vi "Write Outputs.vi"(8 "error in (no error)":errorcluster, 11 "Engine Data in":T1) -> (0 "error out":errorcluster, 3 "Engine Data out":T1)   [LabVIEW 2017, in "Routing and Faulting Engine.lvlib"]
uses:
  Routing and Faulting Engine.lvlib
  Engine Data.ctl
  Includes/CDMessaging.lvlibp/Producer/Abstract Producer/Abstract Producer.lvclass
  Shared/Compiled.Settings.ctl
  Shared/Communication Configuration.ctl
  Shared/Routing and Faulting Configuration.ctl
  Shared/Routing Channel Configuration.ctl
  Shared/Value-Connections Map.ctl
  Shared/Connection.ctl
  Shared/Alias Mapping.ctl
  Shared/FIFO Indices.ctl
  Device Inputs.ctl
  Device Outputs.ctl
  Shared/Routing and Faulting Shared.lvlib
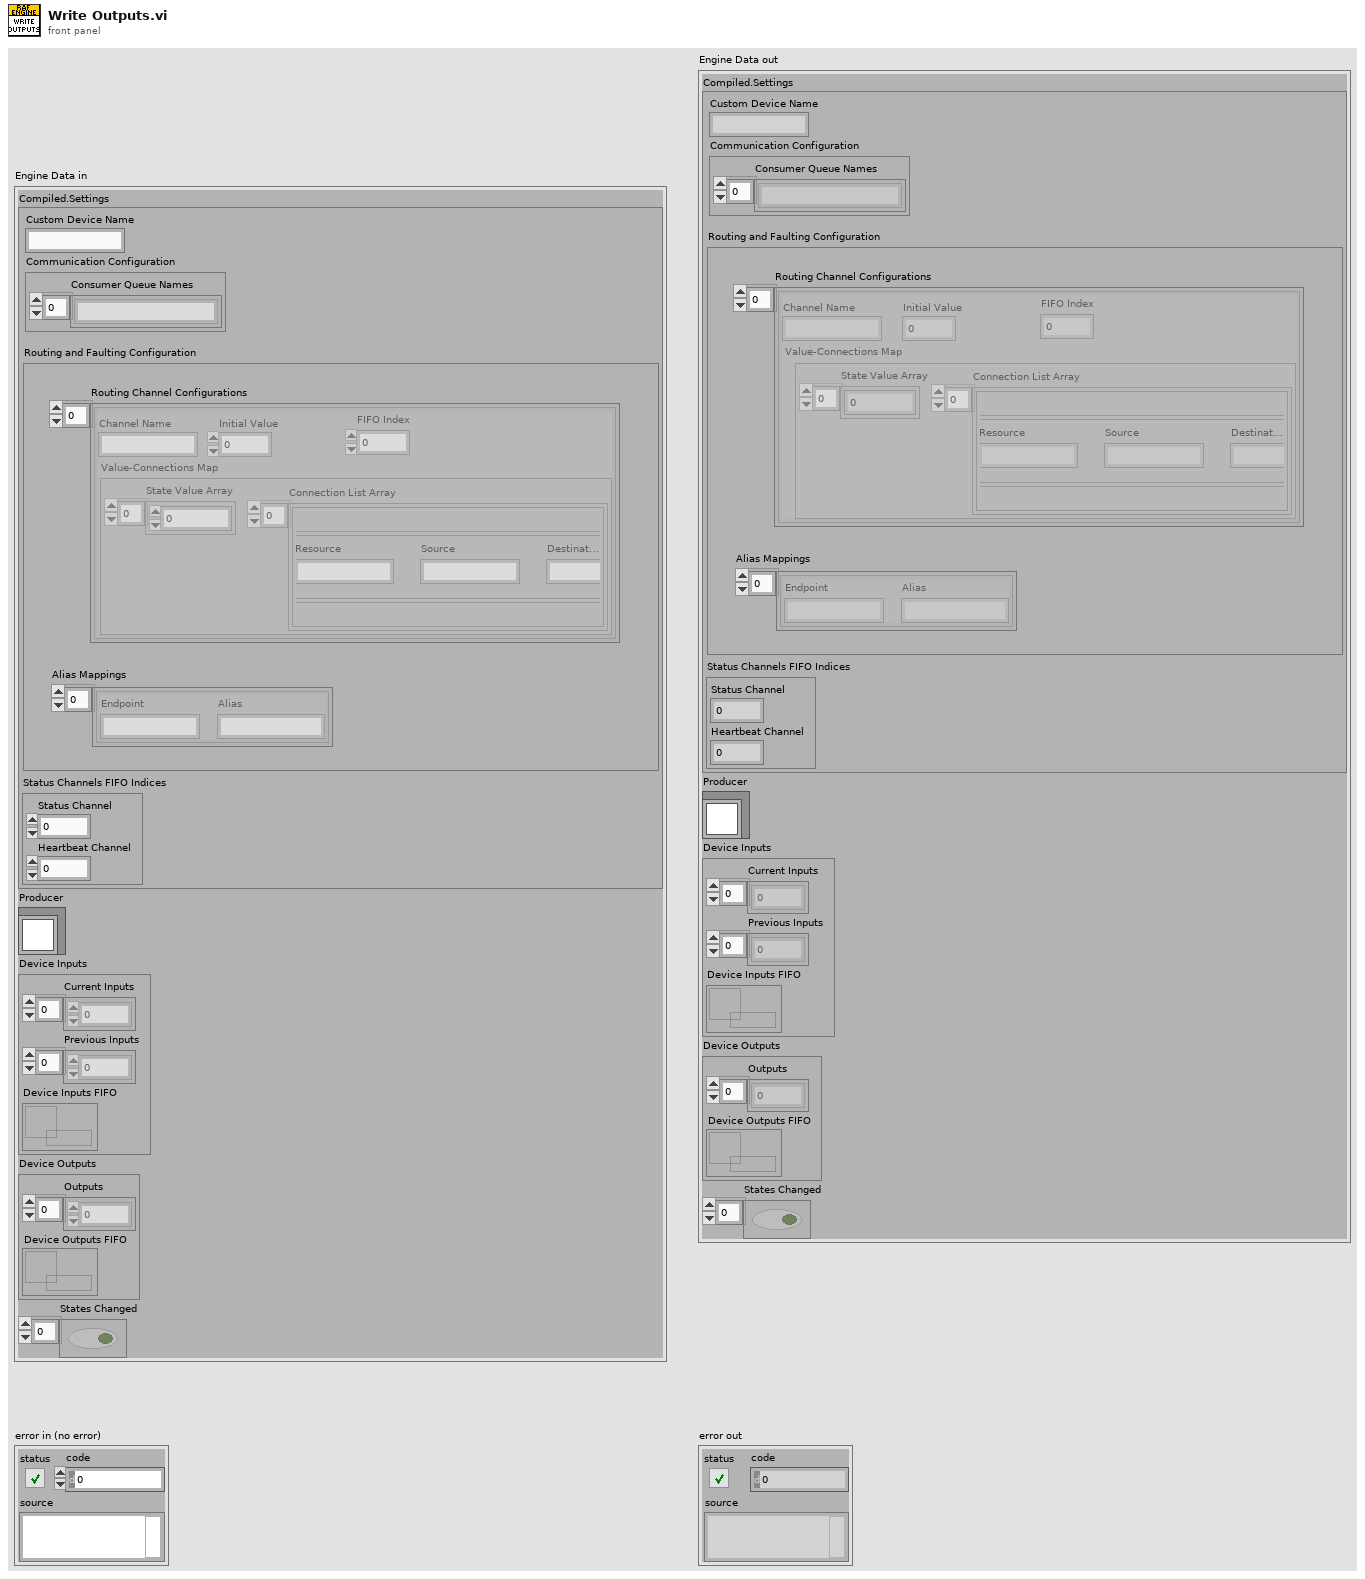
[diagram p1: front panel]
types:
  T1 = typedef "Routing and Faulting Engine.lvlib/Engine Data.ctl" = cluster{"Compiled.Settings":T2, "Producer":refnum<class "Abstract Producer.lvclass">, "Device Inputs":T10, "Device Outputs":T11, "States Changed":bool[]}
  T2 = typedef "Routing and Faulting Shared.lvlib/Compiled.Settings.ctl" = cluster{"Custom Device Name":string, "Communication Configuration":T3, "Routing and Faulting Configuration":T4, "Status Channels FIFO Indices":T9}
  T3 = typedef "Routing and Faulting Shared.lvlib/Communication Configuration.ctl" = cluster{"Consumer Queue Names":string[]}
  T4 = typedef "Routing and Faulting Shared.lvlib/Routing and Faulting Configuration.ctl" = cluster{"Routing Channel Configurations":T5[], "Alias Mappings":T8[]}
  T5 = typedef "Routing and Faulting Shared.lvlib/Routing Channel Configuration.ctl" = cluster{"Channel Name":string, "Initial Value":dbl, "FIFO Index":i32, "Value-Connections Map":T6}
  T6 = typedef "Routing and Faulting Shared.lvlib/Value-Connections Map.ctl" = cluster{"State Value Array":i32[], "Connection List Array":cluster{"Connection List":T7[]}[]}
  T7 = typedef "Routing and Faulting Shared.lvlib/Connection.ctl" = cluster{"Resource":string, "Source":string, "Destination":string}
  T8 = typedef "Routing and Faulting Shared.lvlib/Alias Mapping.ctl" = cluster{"Endpoint":string, "Alias":string}
  T9 = typedef "Routing and Faulting Shared.lvlib/FIFO Indices.ctl" = cluster{"Status Channel":i32, "Heartbeat Channel":i32}
  T10 = typedef "Routing and Faulting Engine.lvlib/Device Inputs.ctl" = cluster{"Current Inputs":dbl[], "Previous Inputs":dbl[], "Device Inputs FIFO":refnum<k33>}
  T11 = typedef "Routing and Faulting Engine.lvlib/Device Outputs.ctl" = cluster{"Outputs":dbl[], "Device Outputs FIFO":refnum<k33>}
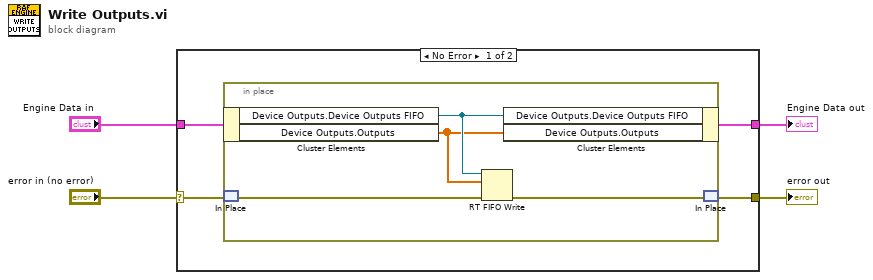
[diagram p0: block diagram]
diagram:
  n1 = case shown="No Error" "error in (no error)" {
    selector: "error in (no error)" -> [w8 w14]
    tunnel: "Engine Data in" -> [w6 w13]
    tunnel: [w7 w14] -> w2
    tunnel: [w5 w13] -> w1
    frame No Error {
      n2 = in-place {
        n3 = in-place-cluster #1(w6) -> ("Device Outputs.Device Outputs FIFO"=w10:refnum<k33>, "Device Outputs.Outputs"=w9:dbl[])
        n4 = in-place-match #2(w8) -> (w12:errorcluster)
        n5 = RT FIFO Write(0:w10, 1:w9, 3:w12) -> (11:w11:errorcluster)  [unwired: 2 in, 3 out]
        n6 = in-place-cluster #1("Device Outputs.Device Outputs FIFO"=w10, "Device Outputs.Outputs"=w9) -> (w5:T1)
        n7 = in-place-match #2(w11) -> (w7:errorcluster)
      }
    }
    frame Error {
    }
  }
  "Engine Data out" <- w1
  "error out" <- w2
